vi "isIncreasing.vi"(9 "End Index":u32, 10 "Start Index":u32, 11 "Array":dbl[](array[numeric])) -> (3 "isIncreasing?":bool)   [LabVIEW 2015]
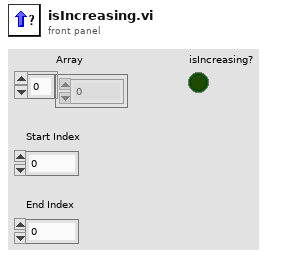
[diagram p1: front panel]
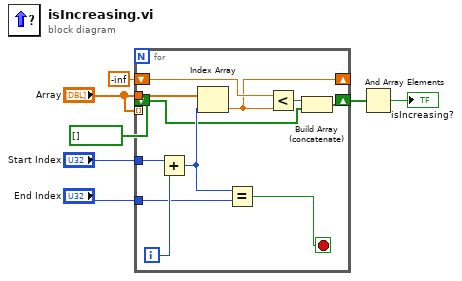
[diagram p0: block diagram]
diagram:
  n1 = for {
    tunnel: "Array" -> [w16]
    tunnel: "Start Index" -> [w18]
    tunnel: "End Index" -> [w14]
    shift-right: [w12] -> _
    shift-left: -inf -> [w13]
    shift-right: [w10] -> w4
    shift-left: bool[] [] -> [w9]
    tunnel: "Array" -> [_] mode=indexing
    i -> [w17]
    stop <- w8 stop-if-true
    n2 = Add(x=w18, y=w17) -> (x+y=w15:u32)
    n3 = Index Array(array=w16, index=w15) -> (element=w12:dbl)
    n4 = Equal?(x=w15, y=w14) -> (x = y?=w8:bool)
    n5 = Less?(x=w13, y=w12) -> (x < y?=w11:bool)
    n6 = Build Array (concatenate)(w11, w9) -> (w10:bool[])
  }
  n7 = And Array Elements(Boolean array=w4) -> (logical AND=→"isIncreasing?":bool)
